vi "Globals.vi"() -> ()   [LabVIEW 2011]
panel:
  in  "Protocols":T1
  in  "Codes":T2
  in  "stop":bool
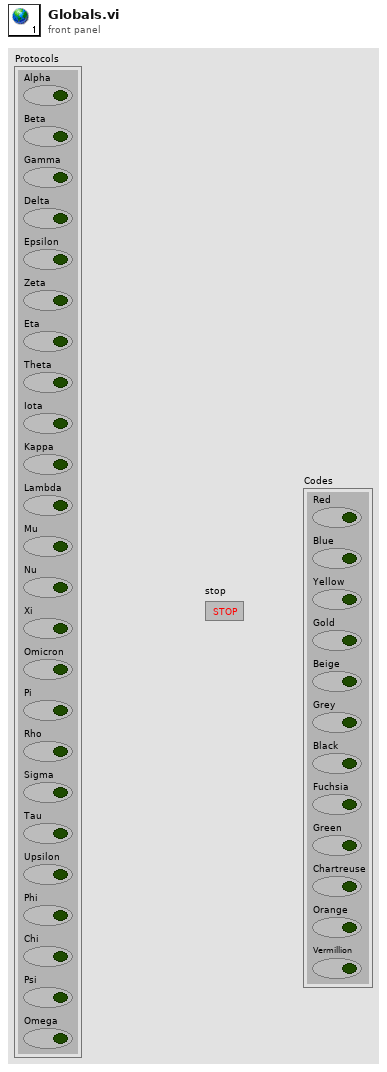
[diagram p1: front panel]
types:
  T1 = cluster{"Alpha":bool, "Beta":bool, "Gamma":bool, "Delta":bool, "Epsilon":bool, "Zeta":bool, "Eta":bool, "Theta":bool, "Iota":bool, "Kappa":bool, "Lambda":bool, "Mu":bool, "Nu":bool, "Xi":bool, "Omicron":bool, "Pi":bool, "Rho":bool, "Sigma":bool, "Tau":bool, "Upsilon":bool, "Phi":bool, "Chi":bool, "Psi":bool, "Omega":bool}
  T2 = cluster{"Red":bool, "Blue":bool, "Yellow":bool, "Gold":bool, "Beige":bool, "Grey":bool, "Black":bool, "Fuchsia":bool, "Green":bool, "Chartreuse":bool, "Orange":bool, "Vermillion":bool}
diagram:
